vi "Configure Measurement.vi"(0 "VISA resource name":refnum<visa-resource-name>, 1 "Ref Level Calculate Method (1:Histogram)":u16(ring)=1 items=["Min-Max", "Histogram", "Histogram Mean"], 2 "Signal Type (0:Pulse)":u16(ring) items=["Pulse", "Eye"], 3 "Eye Noise Measurement (0:Top Level)":u16(ring) items=["Top Level", "Base Level"], 5 "High Ref (90%)":dbl=90.0, 7 "Mid Ref (50%)":dbl=50.0, 9 "Low Ref (10%)":dbl=10.0, 11 "error in (no error)":errorcluster, 12 "Mid2 Ref (50%)":dbl=50.0) -> (4 "VISA resource name out":refnum<visa-resource-name>, 15 "error out":errorcluster)   [LabVIEW 2011, in "Tektronix 7000 Series.lvlib"]
doc: "Configures the reference levels and method an oscilloscope uses to calculate the measurement reference levels. This VI also controls the signal Type."
uses:
  Tektronix 7000 Series.lvlib
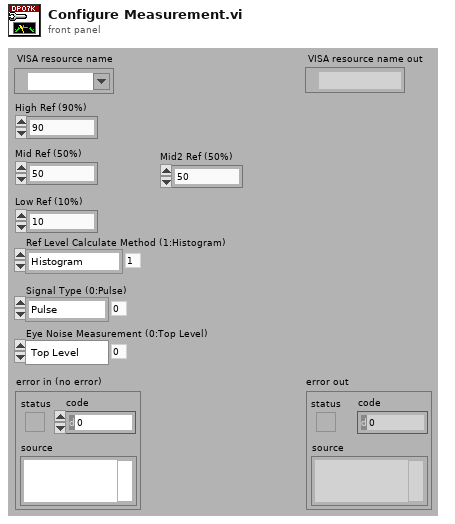
[diagram p1: front panel]
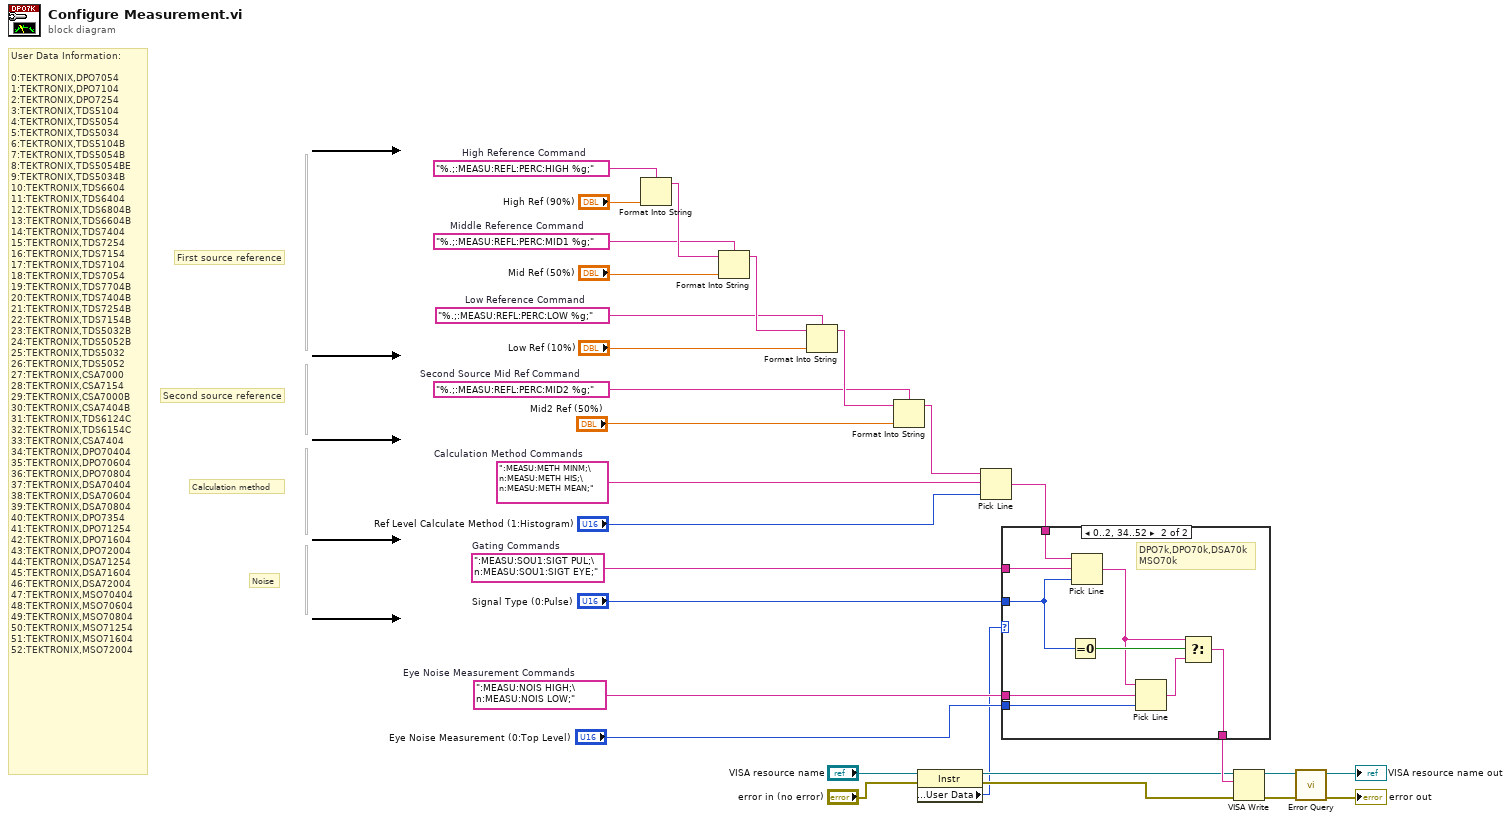
[diagram p0: block diagram]
diagram:
  w7 = ":MEASU:NOIS HIGH;\n:MEASU:NOIS LOW;"  # Eye Noise Measurement Commands
  w17 = ":MEASU:SOU1:SIGT PUL;\n:MEASU:SOU1:SIGT EYE;"  # Gating Commands
  w20 = ":MEASU:METH MINM;\n:MEASU:METH HIS;\n:MEASU:METH MEAN;"  # Calculation Method Commands
  w16 = "%.;:MEASU:REFL:PERC:MID2 %g;"  # Second Source Mid Ref Command
  w22 = "%.;:MEASU:REFL:PERC:LOW %g;"  # Low Reference Command
  w25 = "%.;:MEASU:REFL:PERC:MID1 %g;"  # Middle Reference Command
  w28 = "%.;:MEASU:REFL:PERC:HIGH %g;"  # High Reference Command
  # "User Data Information:\n\n0:TEKTRONIX,DPO7054\n1:TEKTRONIX,DPO7104\n2:TEKTRONIX,DPO7254\n3:TEKTRONIX,TDS5104\n4:TEKTRONIX,TDS5054\n5:TEKTRONIX,TDS5034\n6:TEKTRONIX,TDS5104B\n7:TEKTRONIX,TDS5054B\n8:TEKTRONIX,TDS5054BE\n9:TEKTRONIX,TDS5034B\n10:TEKTRONIX,TDS6604\n11:TEKTRONIX,TDS6404\n12:TEKTRONIX,TDS6804B\n13:TEKTRONIX,TDS6604B\n14:TEKTRONIX,TDS7404\n15:TEKTRONIX,TDS7254\n16:TEKTRONIX,TDS7154\n17:TEKTRONIX,TDS7104\n18:TEKTRONIX,TDS7054\n19:TEKTRONIX,TDS7704B\n20:TEKTRONIX,TDS7404B\n21:TEKTRONIX,TDS7254B\n22:TEKTRONIX,TDS7154B\n23:TEKTRONIX,TDS5032B\n24:TEKTRONIX,TDS5052B\n25:TEKTRONIX,TDS5032\n26:TEKTRONIX,TDS5052\n27:TEKTRONIX,CSA7000\n28:TEKTRONIX,CSA7154\n29:TEKTRONIX,CSA7000B\n30:TEKTRONIX,CSA7404B\n31:TEKTRONIX,TDS6124C\n32:TEKTRONIX,TDS6154C\n33:TEKTRONIX,CSA7404\n34:TEKTRONIX,DPO70404\n35:TEKTRONIX,DPO70604\n36:TEKTRONIX,DPO70804\n37:TEKTRONIX,DSA70404\n38:TEKTRONIX,DSA70604\n39:TEKTRONIX,DSA70804\n40:TEKTRONIX,DPO7354\n41:TEKTRONIX,DPO71254\n42:TEKTRONIX,DPO71604\n43:TEKTRONIX,DPO72004\n44:TEKTRONIX,DSA71254\n45:TEKTRONIX,DSA71604\n46:TEKTRONIX,DSA72004\n47:TEKTRONIX,MSO70404\n48:TEKTRONIX,MSO70604\n49:TEKTRONIX,MSO70804\n50:TEKTRONIX,MSO71254\n51:TEKTRONIX,MSO71604\n52:TEKTRONIX,MSO72004"
  # "Noise"
  # "Calculation method"
  # "Second source reference"
  # "First source reference"
  n1 = Format Into String(format string=w28, "High Ref (90%)") -> (resulting string=w27:string)  [unwired: 2 in, 1 out]
  n2 = Format Into String(format string=w25, initial string=w27, "Mid Ref (50%)") -> (resulting string=w24:string)  [unwired: 1 in, 1 out]
  n3 = Format Into String(format string=w22, initial string=w24, "Low Ref (10%)") -> (resulting string=w21:string)  [unwired: 1 in, 1 out]
  n4 = Format Into String(format string=w16, initial string=w21, "Mid2 Ref (50%)") -> (resulting string=w19:string)  [unwired: 1 in, 1 out]
  n5 = property class="Instr"(reference="VISA resource name", error in="error in (no error)") -> (reference out=w5:refnum<visa-resource-name>, error out=w4:errorcluster, "General Settings:User Data"=w3:u32)
  n6 = Pick Line(string ("")=w19, multi-line string=w20, line index="Ref Level Calculate Method (1:Histogram)") -> (output string=w18:string)
  n7 = case shown="0..2, 34..52" w3 {
    tunnel: w18 -> [w30 w39]
    tunnel: w17 -> [_ w38]
    tunnel: "Signal Type (0:Pulse)" -> [_ w36]
    tunnel: [w30 w35] -> w9
    tunnel: "Eye Noise Measurement (0:Top Level)" -> [_ w33]
    tunnel: w7 -> [_ w32]
    frame Default {
    }
    frame 0..2, 34..52 {
      # "DPO7k,DPO70k,DSA70k\nMSO70k"
      n8 = Equal To 0?(x=w36) -> (x = 0?=w37:bool)
      n9 = Pick Line(string ("")=w39, multi-line string=w38, line index=w36) -> (output string=w34:string)
      n10 = Pick Line(string ("")=w34, multi-line string=w32, line index=w33) -> (output string=w31:string)
      n11 = Select(t=w34, s=w37, f=w31) -> (s? t:f=w35:string)
    }
  }
  n12 = VISA Write(VISA resource name=w5, write buffer=w9, error in (no error)=w4) -> (VISA resource name out=w15:refnum<visa-resource-name>, error out=w14:errorcluster)  [unwired: 1 out]
  n13 = call "Error Query.vi"("error in (no error)"=w14, "VISA resource name"=w15) -> ("error out"=→"error out":errorcluster, "VISA resource name out"=→"VISA resource name out":refnum<visa-resource-name>)  [unwired: 6 in, 2 out]
